vi "updateMode.vi"(8 "error in (no error)":errorcluster, 9 "InternalCommandId.lvclass":refnum<class "InternalCommandId.lvclass">, 10 "Mode":T1, 11 "ElectrometerController in":refnum<class "ElectrometerController.lvclass">) -> (0 "error out":errorcluster, 3 "ElectrometerController out":refnum<class "ElectrometerController.lvclass">)   [LabVIEW 2016, in "ElectrometerController.lvclass"]
uses:
  ElectrometerController.lvclass
  Electrometer/Modes.ctl
  InternalCommandId/InternalCommandId.lvclass
  Electrometer/State/ElectrometerState.lvclass
  Electrometer/Electrometer.lvclass
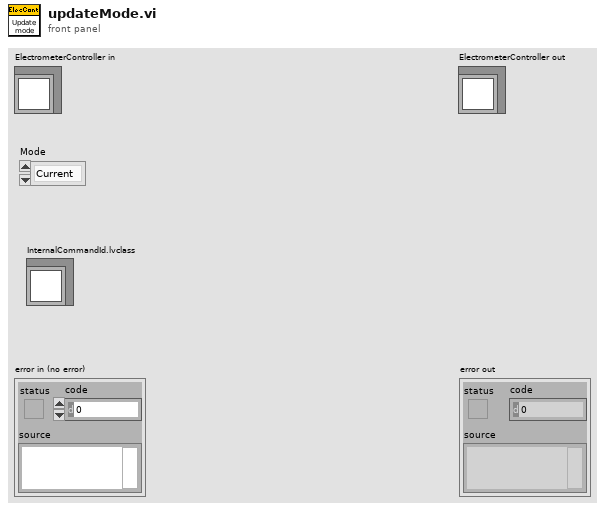
[diagram p1: front panel]
types:
  T1 = typedef "Electrometer.lvclass/Modes.ctl" = enum16{"Current", "Charge"}
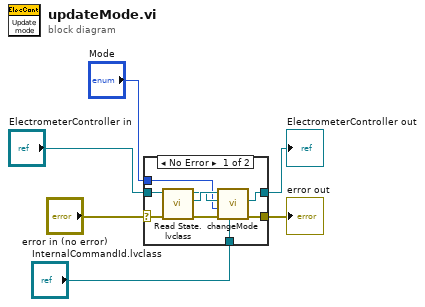
[diagram p0: block diagram]
diagram:
  n1 = case shown="No Error" "error in (no error)" {
    selector: "error in (no error)" -> [w8 w17]
    tunnel: [w12 w17] -> w5
    tunnel: [w11 w16] -> w3
    tunnel: "ElectrometerController in" -> [w9 w16]
    tunnel: "Mode" -> [w10 _]
    tunnel: "InternalCommandId.lvclass" -> [w7 _]
    frame No Error {
      n2 = call-dynamic "Read State.lvclass.vi"("error in (no error)"=w8, "ElectrometerController in"=w9) -> ("error out"=w15:errorcluster, "ElectrometerState"=w14:refnum<class "ElectrometerState.lvclass">, "ElectrometerController out"=w13:refnum<class "ElectrometerController.lvclass">)  [unwired: 7 in]
      n3 = call-dynamic "changeMode.vi"("InternalCommandId.lvclass"=w7, "error in (no error)"=w15, "Mode"=w10, "ElectrometerController in"=w13, "State in"=w14) -> ("error out"=w12:errorcluster, "ElectrometerController out"=w11:refnum<class "ElectrometerController.lvclass">)  [unwired: 4 in, 1 out]
    }
    frame Error {
    }
  }
  "error out" <- w5
  "ElectrometerController out" <- w3
